vi "Read Generated files.vi"(11 "BuildManager in":refnum<class "BuildManager.lvclass">) -> (2 "Generated files":T1[](array[typedef]), 3 "BuildManager out":refnum<class "BuildManager.lvclass">)   [LabVIEW 2019, in "SolutionBuilder.lvlib" / "BuildManager.lvclass"]
uses:
  BuildManager.lvclass
  GeneratedFile.ctl
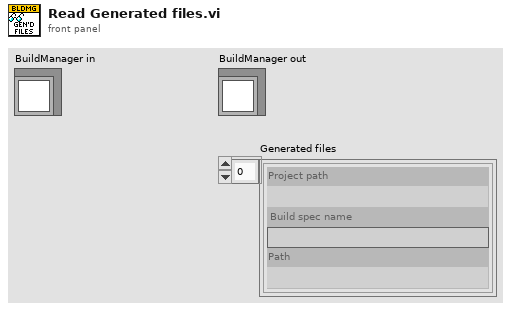
[diagram p1: front panel]
types:
  T1 = typedef "SolutionBuilder.lvlib/BuildManager.lvclass/GeneratedFile.ctl" = cluster{"Project path":path, "Build spec name":string, "Path":path}
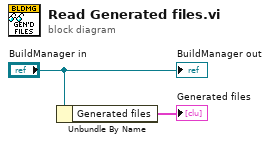
[diagram p0: block diagram]
diagram:
  n1 = Unbundle By Name("BuildManager in") -> ("Generated files"=→"Generated files":T1[])
  "BuildManager out" <- "BuildManager in"
